vi "NML GPIB Data Log Server.vi"() -> ()   [LabVIEW 2020]
uses:
  Sub Controls/NML GPIB List.ctl
panel:
  in  "Seconds":dbl format="%.3e"
  in  "Parameters":dbl[](array[numeric])=[500.0, 1.0, 600.0] caption="Starting Wavelength (nm)\n\nStep (nm)\n\nEnding Wavelength (nm)" format="%.2f"
  in  "Grating Density":u32(ring)=4 items=["150", "300", "600", "1200", "1800"]
  in  "Wait at each Step":T2={"Instrument"=enum."Time Stamp", "GPIB Address"=1, "(Seconds)"=[1.0]} {"(Seconds)" format="%.3e"; "GPIB Address" min=1 max=31 step=1}
  in  "McPherson Spectrometer Parameters":T3={"Instrument"=enum."IMS Stepper Increment", "Grating Density"=4, "Parameters"=[500.0, 1.0, 600.0]} {"Parameters" format="%.2f"; "Grating Density" items=["150", "300", "600", "1200", "1800"]}
  in  "Culster":T4={"McPherson Spectrometer Parameters"={"Instrument"=enum."IMS Stepper Increment", "Grating Density"=4, "Parameters"=[500.0, 1.0, 600.0]}, "Wait at each Step"={"Instrument"=enum."Time Stamp", "GPIB Address"=1, "(Seconds)"=[1.0]}, "#1"={"Instrument"=enum."None", "GPIB Address"=5, "Parameters"=[]}, "#2"={"Instrument"=enum."None", "GPIB Address"=6, "Parameters"=[]}, "#3"={"Instrument"=enum."None", "GPIB Address"=7, "Parameters"=[]}, "#4"={"Instrument"=enum."None", "GPIB Address"=8, "Parameters"=[]}, "#5"={"Instrument"=enum."None", "GPIB Address"=9, "Parameters"=[]}, "#6"={"Instrument"=enum."None", "GPIB Address"=10, "Parameters"=[]}, "#7"={"Instrument"=enum."None", "GPIB Address"=11, "Parameters"=[]}, "#8"={"Instrument"=enum."None", "GPIB Address"=12, "Parameters"=[]}} {"#8"."Parameters" format="%.3e"; "#8"."GPIB Address" min=1 max=31 step=1; "#7"."Parameters" format="%.3e"; "#7"."GPIB Address" min=1 max=31 step=1; "#6"."Parameters" format="%.3e"; "#6"."GPIB Address" min=1 max=31 step=1; "#5"."Parameters" format="%.3e"; "#5"."GPIB Address" min=1 max=31 step=1; "#4"."Parameters" format="%.3e"; "#4"."GPIB Address" min=1 max=31 step=1; "#3"."Parameters" format="%.3e"; "#3"."GPIB Address" min=1 max=31 step=1; "#2"."Parameters" format="%.3e"; "#2"."GPIB Address" min=1 max=31 step=1; "#1"."Parameters" format="%.3e"; "#1"."GPIB Address" min=1 max=31 step=1; "McPherson Spectrometer Parameters"."Parameters" format="%.2f"; "McPherson Spectrometer Parameters"."Grating Density" items=["150", "300", "600", "1200", "1800"]; "Wait at each Step"."(Seconds)" format="%.3e"; "Wait at each Step"."GPIB Address" min=1 max=31 step=1}
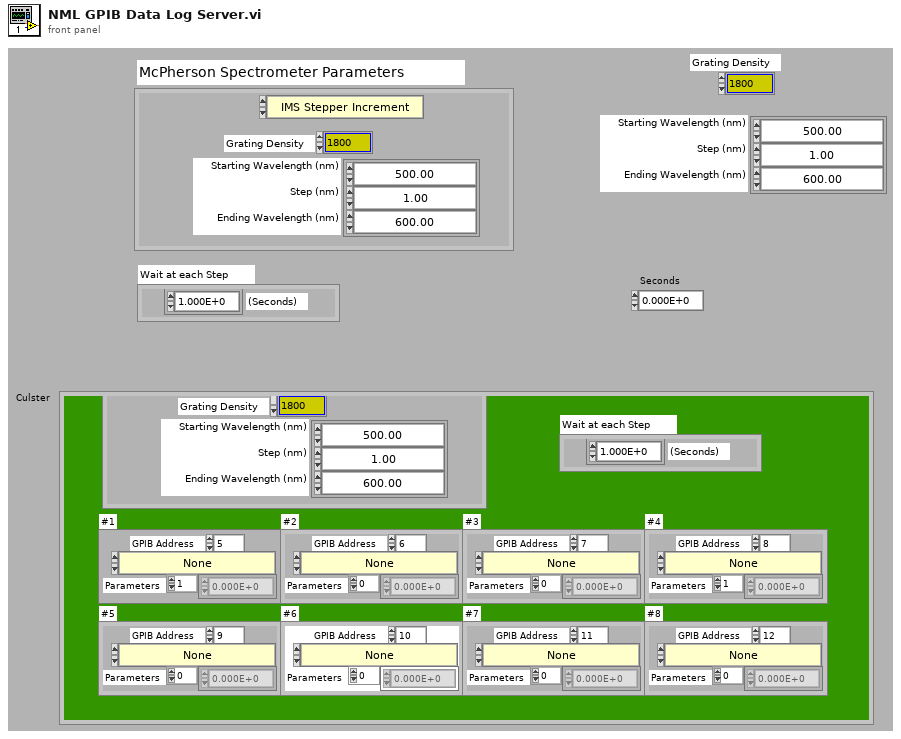
[diagram p1: front panel]
types:
  T1 = typedef "NML GPIB List.ctl" = enum16{"None", "Field", "Field - SCM1", "DMM", "DMM - HP 34401", "Keithley 2XXX", "Running DMM Ave", "Running HP34401", "Running K2XXX Ave", "SRS 830 - CH 1", "SRS 830 - CH1 & 2", "SRS PTC10", "Signal Rec 7265 - X", "Signal Rec 7265 - X&Y", "DRC 93C - Sample", "DRC 93C - Control", "DRC 93C - Sam&Con", "CryoCon Sensor A", "CryoCon Sensor B", "Cond 20C Sensor 1", "Cond 20C Sensor 2", "LS 336 Read", "LS 340 Read", "LS 370 Read", "LS 370 Select", "AVS 46 Bridge", "BLM Rotator Read Position", "Linear Research 700", "LR 700 Select", "Keithley 3330 - LCZ", "A-H Capacitance", "Digital Integrator", "SRS 400 Phot Ctr", "LakeShore VSM", "AMI He Level Meter", "Time Stamp", "Wait", "Invert Current", "K230 Linear V", "K230 VÅB^2", "Temp Ramp", "Power Ramp", "Freq Sweep", "LTC Stable T", "Scanner Step", "IMS Stepper Increment", "BLM Stepper Increment", "Omega CNi32"}
  T2 = cluster{"Instrument":T1, "GPIB Address":u32, "(Seconds)":dbl[]}
  T3 = cluster{"Instrument":T1, "Grating Density":u32, "Parameters":dbl[]}
  T4 = cluster{"McPherson Spectrometer Parameters":cluster{"Instrument":T1, "Grating Density":u32, "Parameters":dbl[]}, "Wait at each Step":cluster{"Instrument":T1, "GPIB Address":u32, "(Seconds)":dbl[]}, "#1":cluster{"Instrument":T1, "GPIB Address":u32, "Parameters":dbl[]}, "#2":cluster{"Instrument":T1, "GPIB Address":u32, "Parameters":dbl[]}, "#3":cluster{"Instrument":T1, "GPIB Address":u32, "Parameters":dbl[]}, "#4":cluster{"Instrument":T1, "GPIB Address":u32, "Parameters":dbl[]}, "#5":cluster{"Instrument":T1, "GPIB Address":u32, "Parameters":dbl[]}, "#6":cluster{"Instrument":T1, "GPIB Address":u32, "Parameters":dbl[]}, "#7":cluster{"Instrument":T1, "GPIB Address":u32, "Parameters":dbl[]}, "#8":cluster{"Instrument":T1, "GPIB Address":u32, "Parameters":dbl[]}}
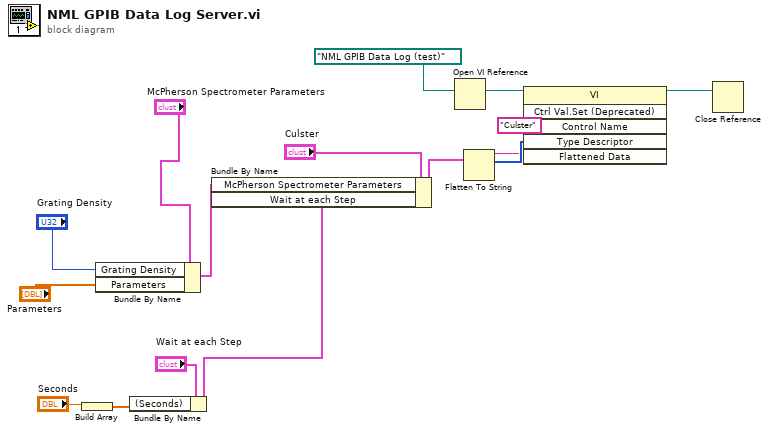
[diagram p0: block diagram]
diagram:
  n1 = Build Array("Seconds") -> (w1:dbl[])
  n2 = Bundle By Name(cluster="McPherson Spectrometer Parameters", "Grating Density"="Grating Density", "Parameters"="Parameters") -> (w5:T3)
  n3 = Bundle By Name(cluster="Wait at each Step", "(Seconds)"=w1) -> (w3:T2)
  n4 = Bundle By Name(cluster="Culster", "McPherson Spectrometer Parameters"=w5, "Wait at each Step"=w3) -> (w9:T4)
  n5 = Open VI Reference(vi path=path "NML GPIB Data Log (test)") -> (vi reference=w15:refnum<vi>)  [unwired: 5 in, 1 out]
  n6 = Flatten To String(anything=w9) -> (data string=w11:string, type string=w12:i16[])  [unwired: 3 in, 1 out]
  n7 = invoke class="VI" method="Ctrl Val.Set (Deprecated)"(reference=w15, "Control Name"="Culster", "Type Descriptor"=w12, "Flattened Data"=w11) -> (reference out=w14:refnum<vi>)  [unwired: 2 in, 5 out]
  n8 = Close Reference(reference=w14) -> ()  [unwired: 1 in, 1 out]
